vi "RIGOLfix.vi"(10 "Amplitude (Vpp)":dbl=1.0, 11 "Frequency (MHz)":dbl=85.0) -> ()   [LabVIEW 2012]
uses:
  <vilib>/Instr/_visa.llb/VISA Open Access Mode.ctl
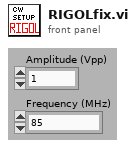
[diagram p1: front panel]
types:
  T1 = typedef "VISA Open Access Mode.ctl" = u32
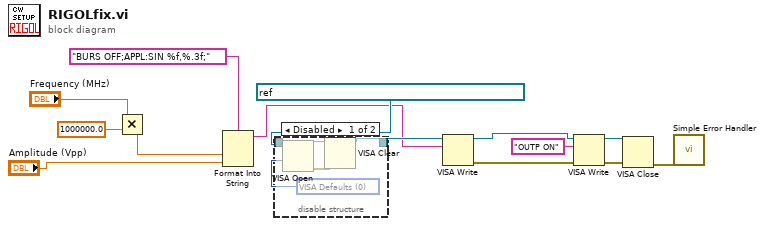
[diagram p0: block diagram]
diagram:
  n1 = Multiply(x="Frequency (MHz)", y=1000000.0) -> (x*y=w11:dbl)
  n2 = Format Into String(format string="BURS OFF;APPL:SIN %f,%.3f;", w11, "Amplitude (Vpp)") -> (resulting string=w1:string)  [unwired: 2 in, 1 out]
  n3 = disable-structure shown="Disabled" {
    disable-tunnel: [w19 w20] -> w6
    disable-tunnel: refnum<visa-resource-name> "USB0::0x1AB1::0x0641::DG4B142100247::INSTR" ("VISA resource name") -> [w18 w20]
    frame Disabled {
      w16 = T1 0 items=["VISA Defaults"=0, "Exclusive Lock"=1, "Load Configured Settings"=4] ("Access Mode")
      n4 = VISA Open(access mode=w16, VISA resource name=w18) -> (VISA resource name=w17:refnum<visa-resource-name>, error out=w15:errorcluster)  [unwired: 3 in]
      n5 = VISA Clear(VISA resource name=w17, error in (no error)=w15) -> (VISA resource name out=w19:refnum<visa-resource-name>)  [unwired: 1 out]
    }
    frame Enabled {
    }
  }
  n6 = VISA Write(VISA resource name=w6, write buffer=w1) -> (VISA resource name out=w7:refnum<visa-resource-name>, error out=w8:errorcluster)  [unwired: 1 in, 1 out]
  n7 = VISA Write(VISA resource name=w7, write buffer="OUTP ON", error in (no error)=w8) -> (VISA resource name out=w4:refnum<visa-resource-name>, error out=w3:errorcluster)  [unwired: 1 out]
  n8 = VISA Close(VISA resource name=w4, error in (no error)=w3) -> (error out=w2:errorcluster)
  n9 = call <vilib>:"Simple Error Handler.vi"("error in (no error)"=w2) -> ()  [unwired: 4 in, 5 out]
